vi "generate run flag.vi"(11 "execution settings":T1) -> (3 "run flags":u8)   [LabVIEW 2013, in "Standard Engine Runtime.lvclass"]
uses:
  Standard Engine Runtime.lvclass
  <vilib>/NI/Tag Bus Module Framework/runtime/execution settings.ctl
  <vilib>/NI/Tag Bus Module Framework/runtime/TBM module execution interface.lvclass
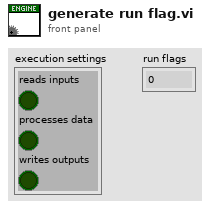
[diagram p1: front panel]
types:
  T1 = typedef "TBM module execution interface.lvclass/execution settings.ctl" = cluster{"reads inputs":bool, "processes data":bool, "writes outputs":bool}
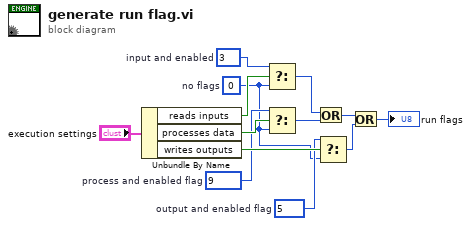
[diagram p0: block diagram]
diagram:
  w6 = u8 0  # no flags
  w7 = u8 9  # process and enabled flag
  w8 = u8 5  # output and enabled flag
  w9 = u8 3  # input and enabled
  n1 = Unbundle By Name("execution settings") -> ("reads inputs"=w12:bool, "processes data"=w11:bool, "writes outputs"=w10:bool)
  n2 = Select(t=w9, s=w12, f=w6) -> (s? t:f=w5:u8)
  n3 = Select(t=w7, s=w11, f=w6) -> (s? t:f=w4:u8)
  n4 = Or(x=w5, y=w4) -> (x .or. y?=w3:u8)
  n5 = Select(t=w8, s=w10, f=w6) -> (s? t:f=w2:u8)
  n6 = Or(x=w3, y=w2) -> (x .or. y?=→"run flags":u8)
